vi "think_and_act_2.vi"(8 "error in (no error)":errorcluster, 9 "antState":T1, 10 "pieceOfWorld":T4[][](array[typedef]), 11 "Igor in":refnum<class "Igor.lvclass">) -> (0 "error out":errorcluster, 2 "action":T2, 3 "Igor out":refnum<class "Igor.lvclass">)   [LabVIEW 2015]
doc: "Ant thinks and chooses action\nCreated by Artem Shevelev\nshevelev.pro\nartem@shevelev.pro\nLabVIEW Portal: https://labviewportal.org/memberlist.php?mode=viewprofile&u=2340"
uses:
  ant_base/ant_base.lvclass
  ant_base/actionType_enum.ctl
  ant_base/action_cluster.ctl
  actors/world/typedefs/markValue.ctl
  actors/world/world.lvlib
  actors/world/typedefs/anthillType_enum.ctl
  Igor.lvclass
  az_to_rad/az_to_rad_back.vi
  az_to_rad/az_to_rad_straight.vi
  actors/world/typedefs/markVolume.ctl
  actors/world/typedefs/markValue_cluster.ctl
  actors/world/typedefs/worldCell_cluster.ctl
  ant_base/antState_cluster.ctl
  actors/world/typedefs/amountOfFood.ctl
panel:
  out "Array":i32[][](array[numeric])
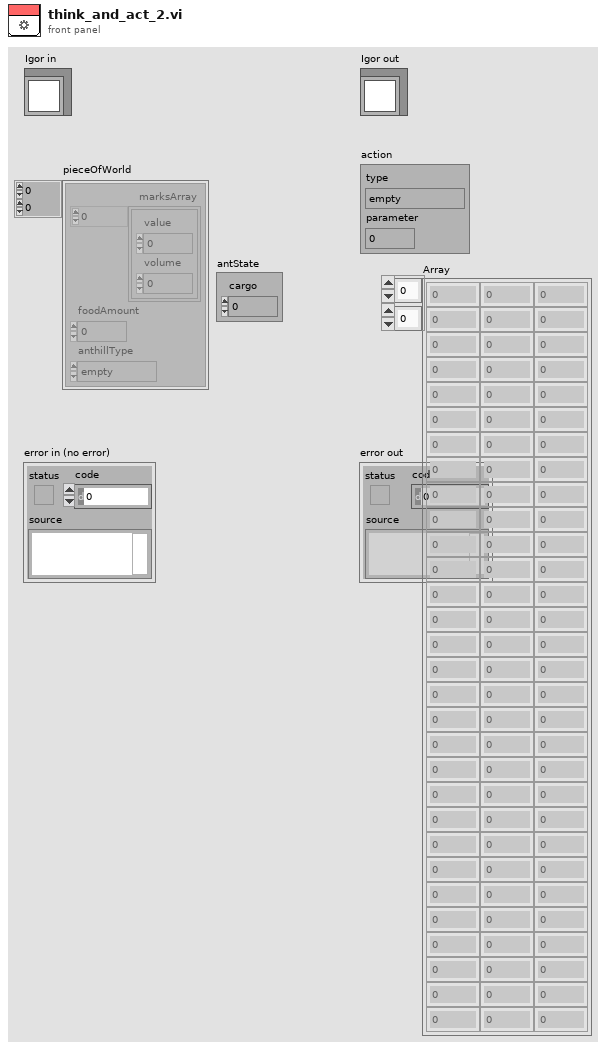
[diagram p1: front panel]
types:
  T1 = typedef "ant_base.lvclass/antState_cluster.ctl" = cluster{"cargo":u8}
  T2 = typedef "ant_base.lvclass/action_cluster.ctl" = cluster{"type":T3, "parameter":dbl}
  T3 = typedef "ant_base.lvclass/actionType_enum.ctl" = enum8{"empty", "move", "take", "put", "mark"}
  T4 = typedef "world.lvlib/worldCell_cluster.ctl" = cluster{"marksArray":T5[], "foodAmount":T8, "anthillType":T9}
  T5 = typedef "world.lvlib/markValue_cluster.ctl" = cluster{"value":T6, "volume":T7}
  T6 = typedef "world.lvlib/markValue.ctl" = u8
  T7 = typedef "world.lvlib/markVolume.ctl" = u16
  T8 = typedef "world.lvlib/amountOfFood.ctl" = i32
  T9 = typedef "world.lvlib/anthillType_enum.ctl" = enum16{"empty", "own", "rival"}
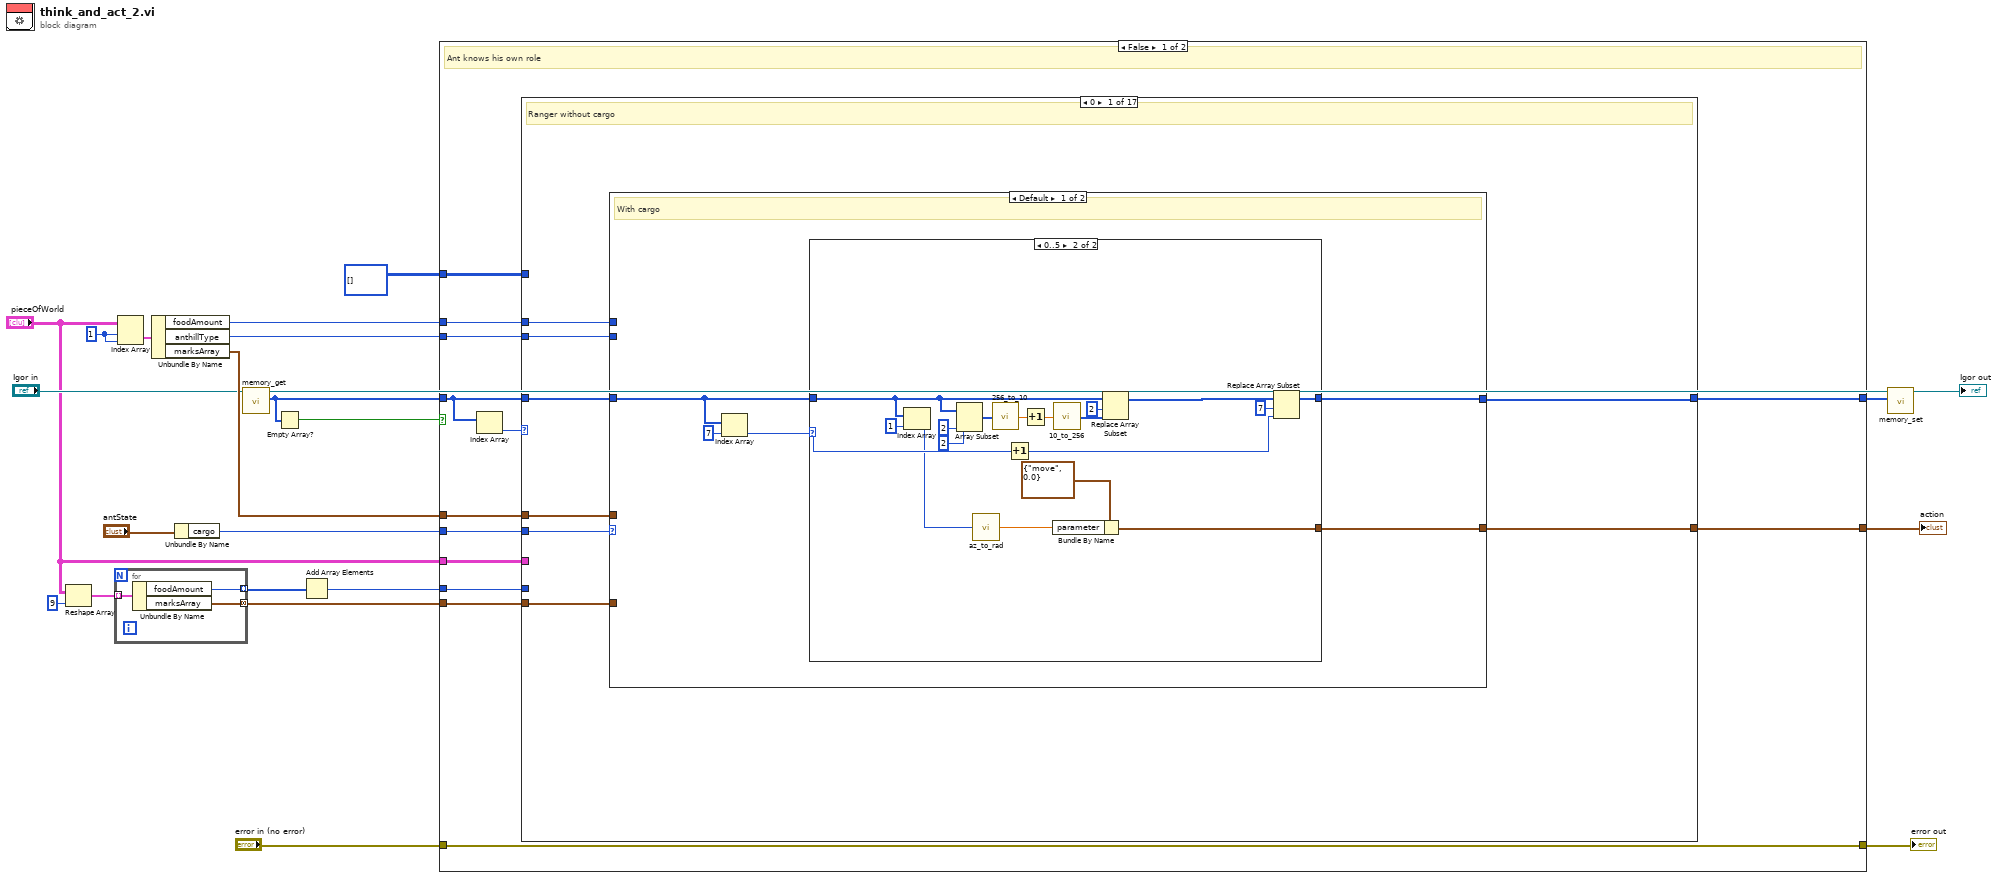
[diagram p0: block diagram]
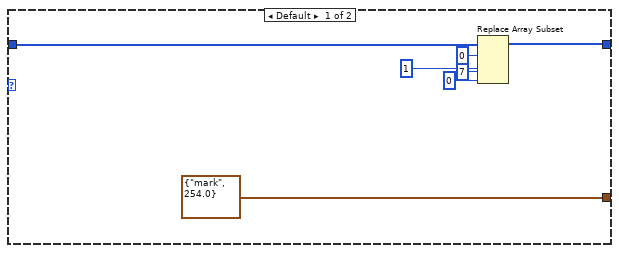
[diagram p2: hidden frame]
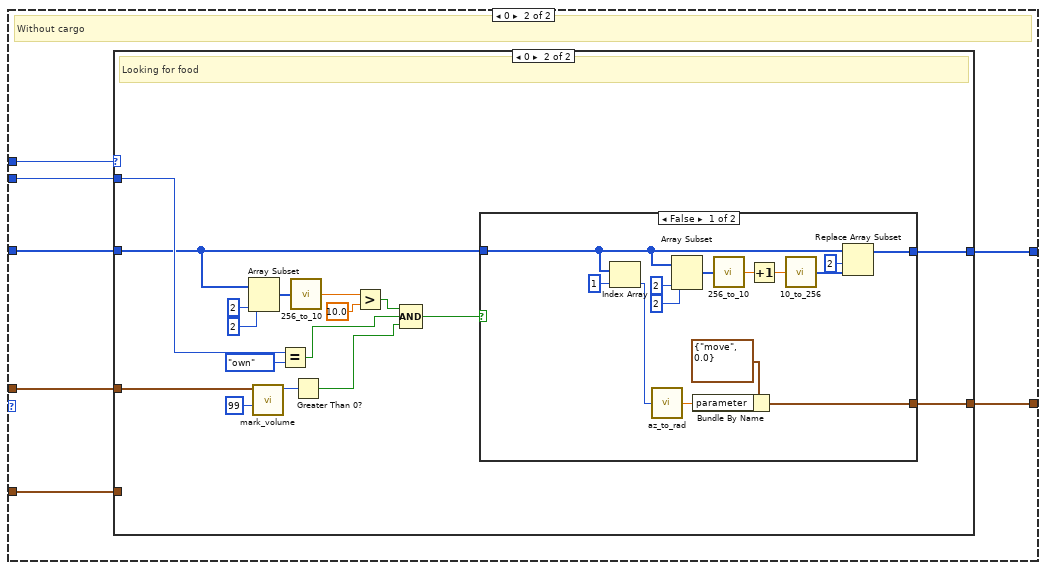
[diagram p3: hidden frame]
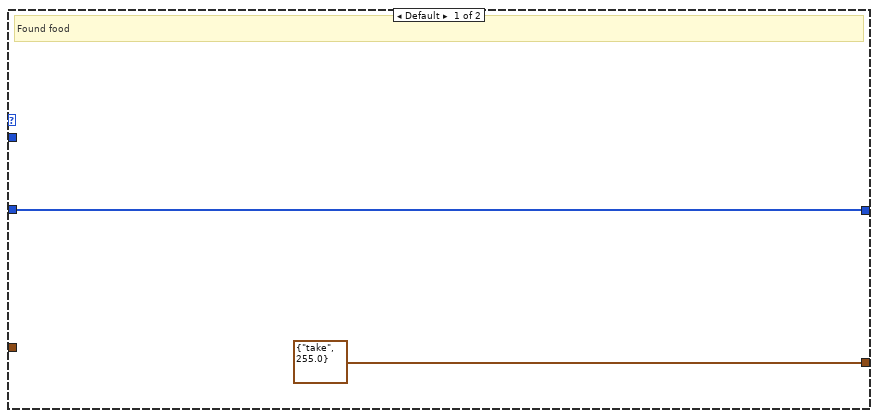
[diagram p4: hidden frame]
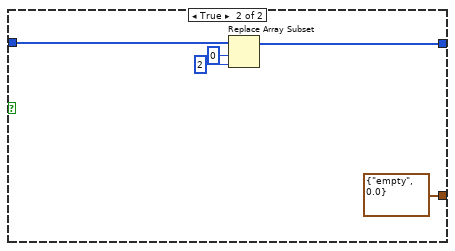
[diagram p5: hidden frame]
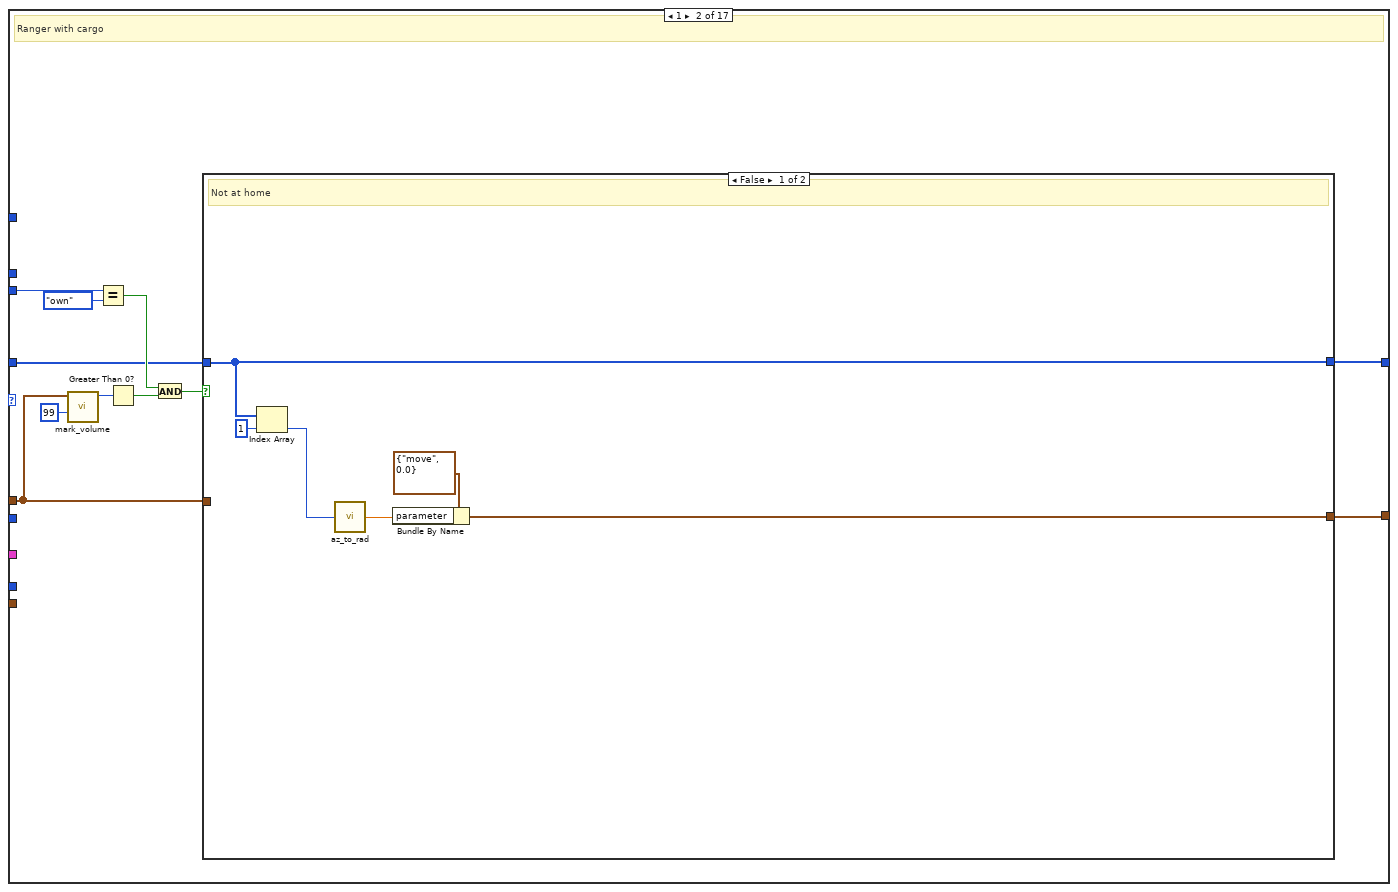
[diagram p6: hidden frame]
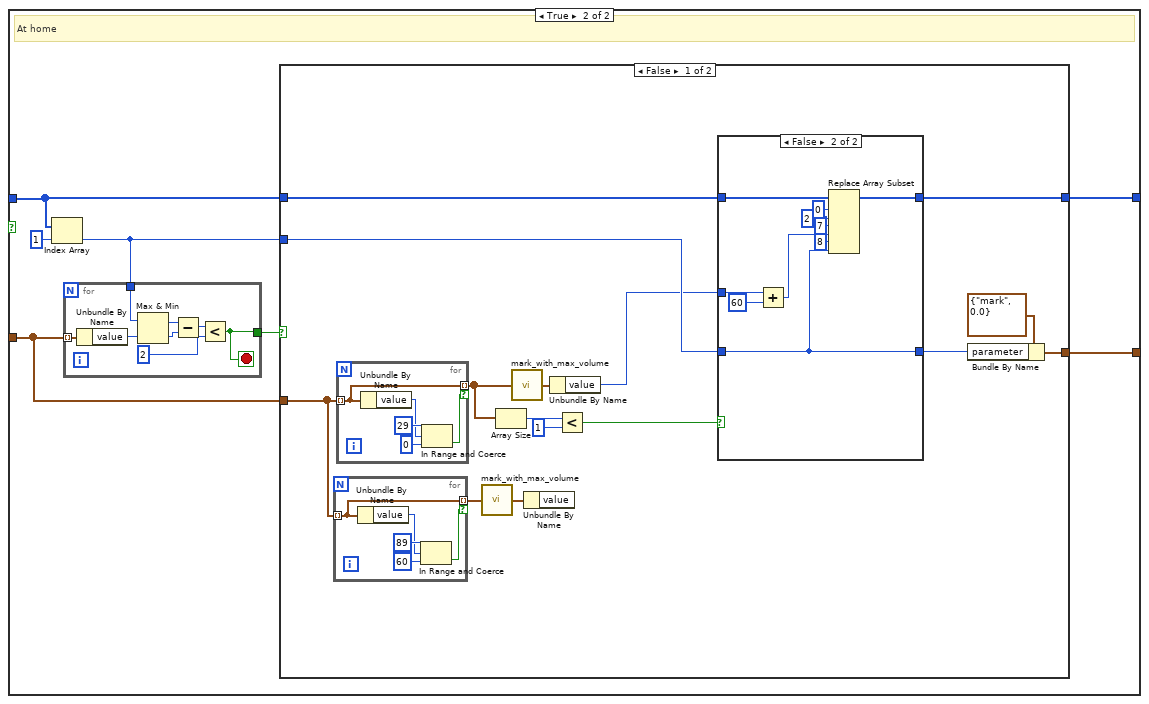
[diagram p7: hidden frame]
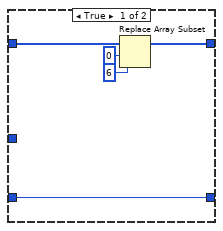
[diagram p8: hidden frame]
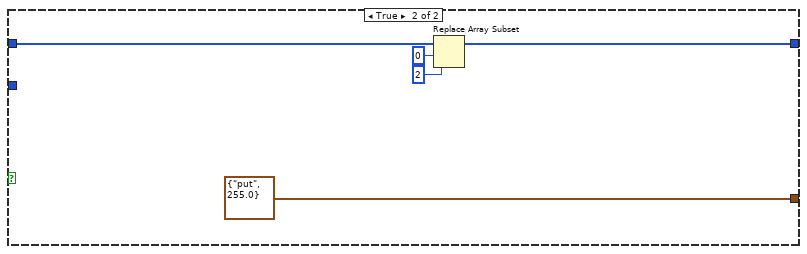
[diagram p9: hidden frame]
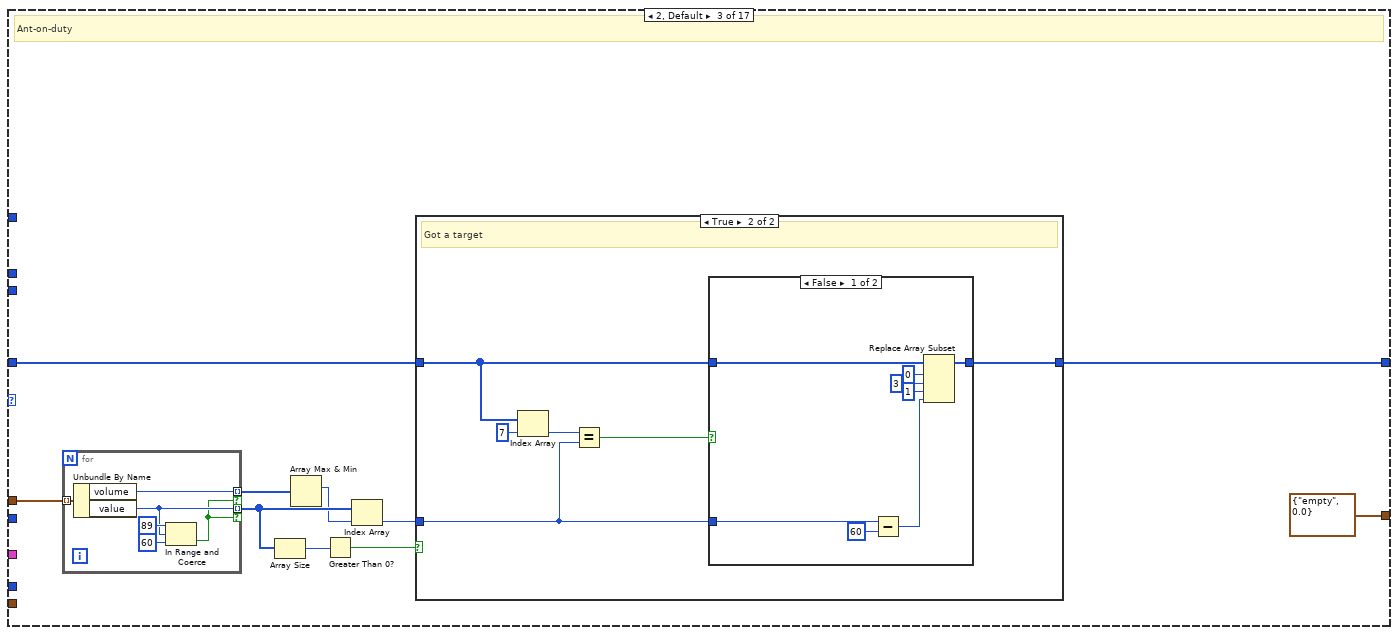
[diagram p10: hidden frame]
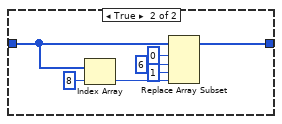
[diagram p12: hidden frame]
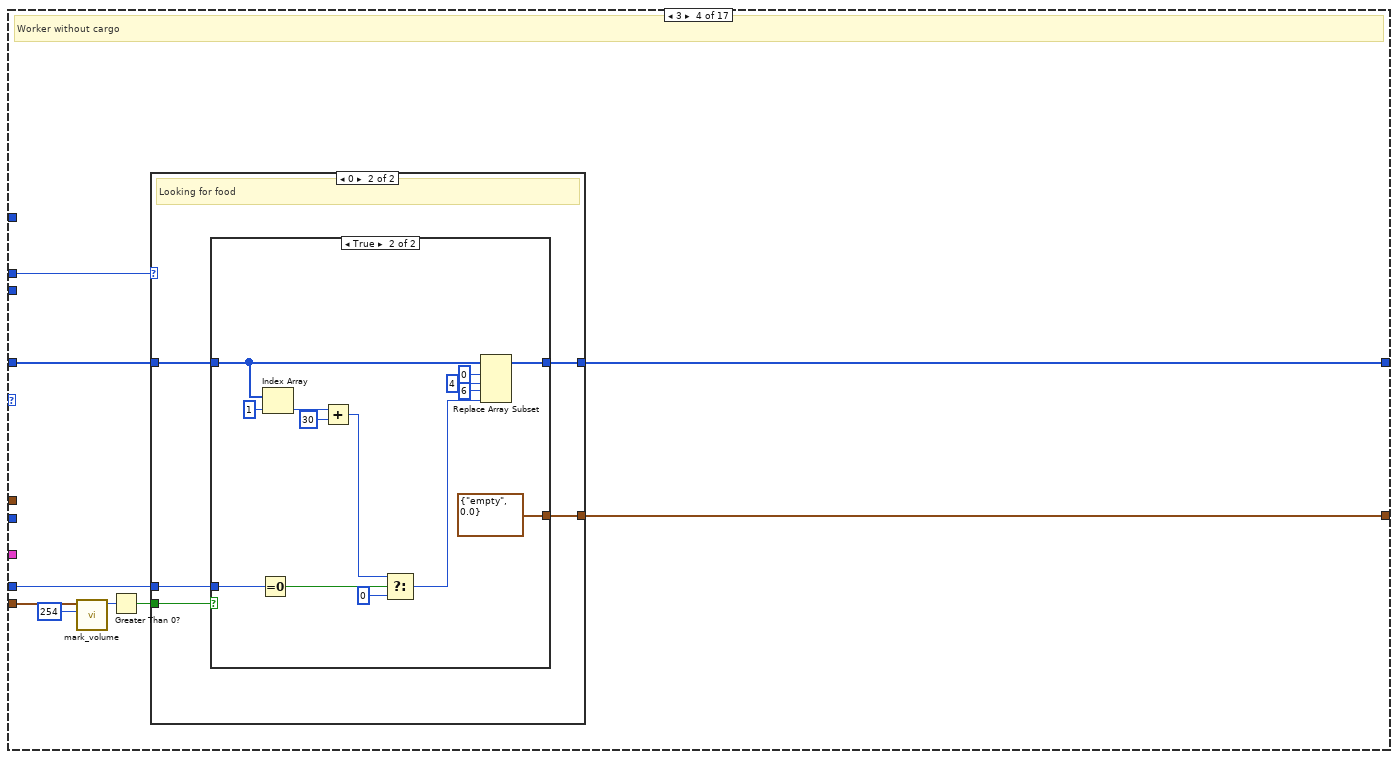
[diagram p13: hidden frame]
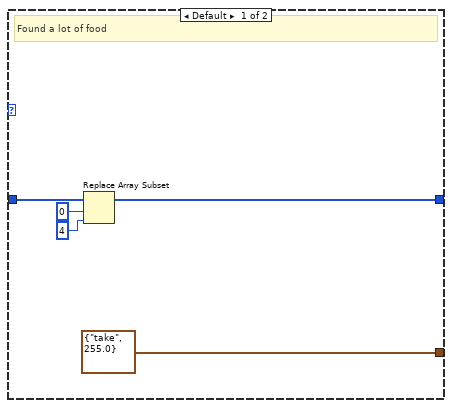
[diagram p14: hidden frame]
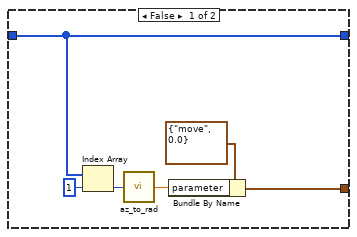
[diagram p15: hidden frame]
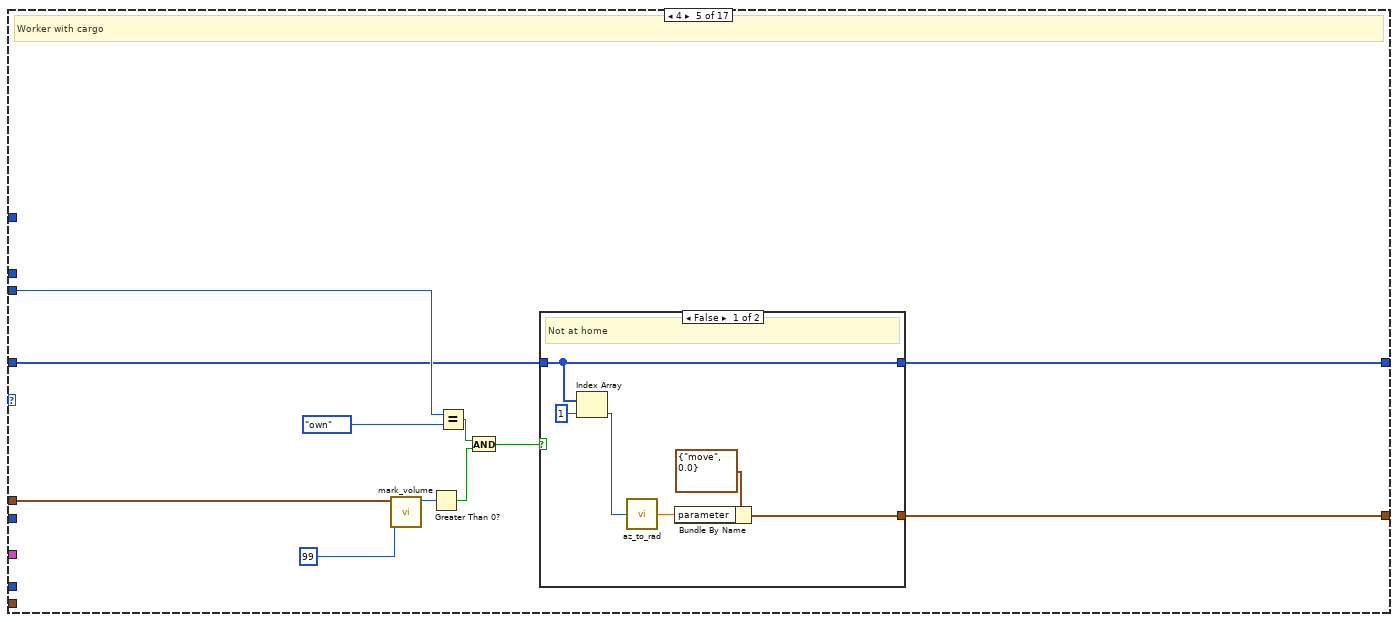
[diagram p16: hidden frame]
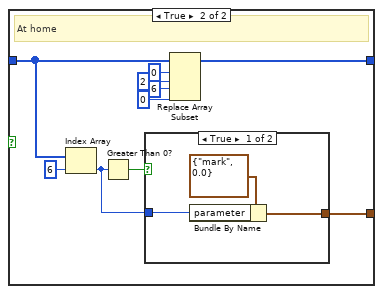
[diagram p17: hidden frame]
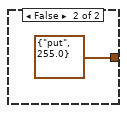
[diagram p18: hidden frame]
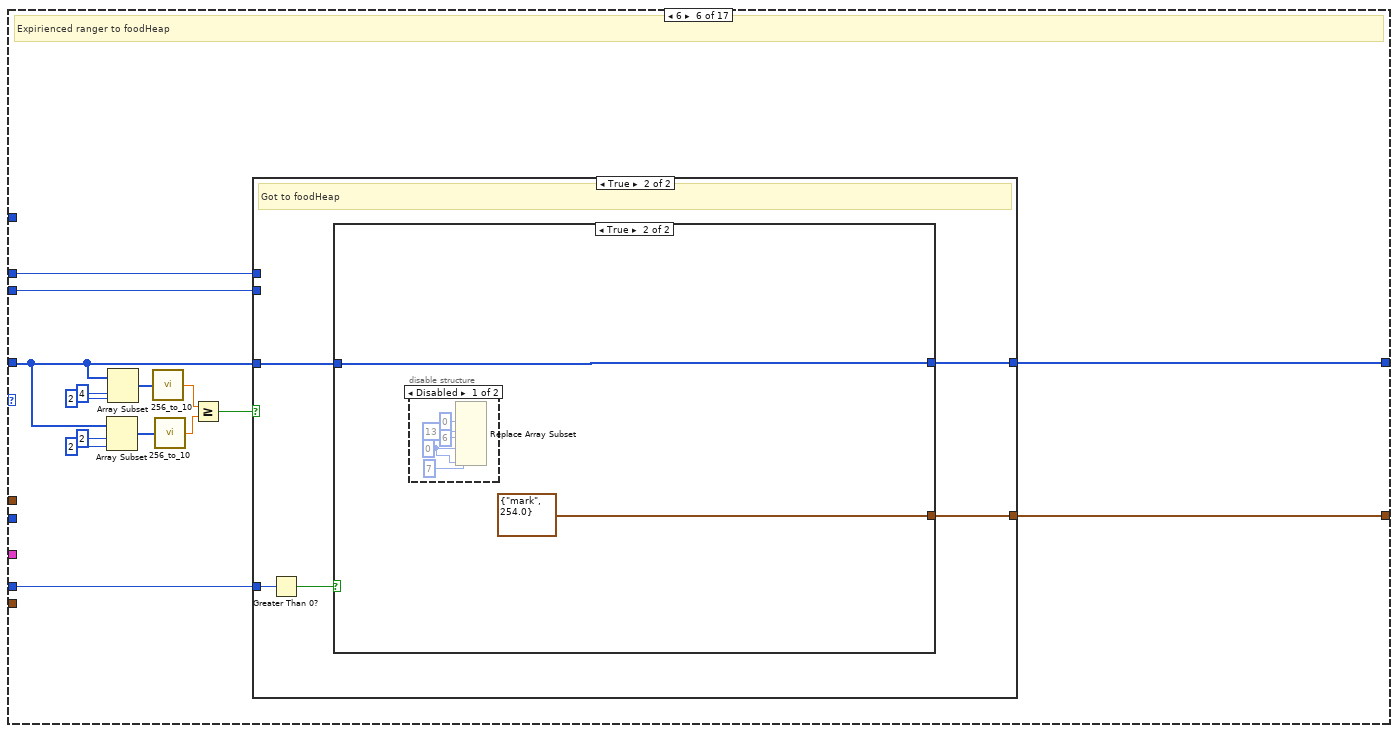
[diagram p19: hidden frame]
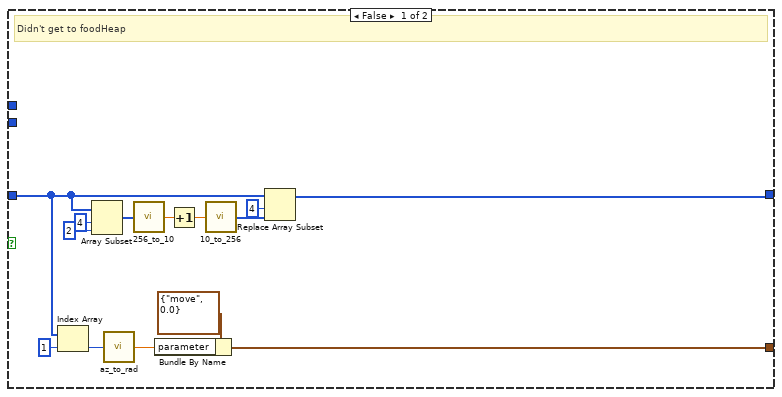
[diagram p20: hidden frame]
diagram:
  w23 = 1 ("index (row)")
  n1 = Reshape Array("pieceOfWorld", 9 ("dimension size")) -> (w10:T4[])
  n2 = for {
    tunnel: w10 -> [w26] mode=indexing
    tunnel: [w25] -> w9 mode=concatenating
    tunnel: [w24] -> w8 mode=indexing
    n3 = Unbundle By Name(w26) -> ("foodAmount"=w24:T8, "marksArray"=w25:T5[])
  }
  n4 = Index Array(array="pieceOfWorld", index (row)=w23, index (col)=w23) -> (element=w22:T4)
  n5 = Unbundle By Name(w22) -> ("foodAmount"=w14:T8, "anthillType"=w13:T9, "marksArray"=w18:T5[])
  n6 = Unbundle By Name("antState") -> ("cargo"=w2:u8)
  n7 = call "memory_get.vi"("ant_base in"="Igor in") -> ("memory"=w15:u8[], "ant_base out"=w5:refnum<class "Igor.lvclass">)  [unwired: 8 in, 1 out]
  n8 = Empty Array?(array=w15) -> (empty?=w16:bool)
  n9 = Add Array Elements(numeric array=w8) -> (sum=w7:T8)
  n10 = case shown="False" w16 {
    tunnel: [w39 w791] -> w21
    tunnel: [w37 w790] -> w20
    tunnel: "error in (no error)" -> [w39 w791]
    tunnel: w18 -> [w34 w786]
    tunnel: w15 -> [w33 w787]
    tunnel: w14 -> [w36 _]
    tunnel: w13 -> [w35 _]
    tunnel: "pieceOfWorld" -> [w32 _]
    tunnel: w9 -> [w31 _]
    tunnel: w7 -> [w30 _]
    tunnel: [w29 w788] -> w4
    tunnel: w2 -> [w28 _]
    tunnel: i32[][] [] -> [w27 _]
    frame False {
      # "Ant knows his own role"
      n11 = Index Array(array=w33) -> (element=w38:u8)  [unwired: 1 in]
      n12 = case shown="0" w38 {
        tunnel: [w47 w133 T2 {"type"=enum."empty", "parameter"=0.0} ("action") w245 w286 w313 w365 w409 T2 {"type"=enum."empty", "parameter"=0.0} ("action") w433 T2 {"type"=enum."empty", "parameter"=0.0} ("action") w525 w548 w575 w612 w637 w685] -> w37
        tunnel: w36 -> [w46 _ _ w239 _ w314 _ _ _ w430 _ _ _ _ w613 _ _]
        tunnel: w35 -> [w44 w132 _ _ w287 w311 w367 _ _ w431 _ _ _ w574 w611 w639 _]
        tunnel: w34 -> [w41 w126 w209 _ w279 _ w359 w400 _ _ w473 _ _ w568 w608 w632 w678]
        tunnel: w33 -> [w45 w128 w201 w246 w285 w315 w366 w410 w427 w435 w487 w524 w547 w570 w614 w638 w684]
        tunnel: w32 -> [_ _ _ _ _ _ _ _ _ _ _ _ _ _ _ _ _]
        tunnel: w31 -> [w43 _ _ w240 _ _ _ _ _ _ _ _ _ _ _ _ _]
        tunnel: w30 -> [_ _ _ w238 _ w310 _ _ _ _ _ _ _ _ w610 _ _]
        tunnel: [w42 w123 w200 w241 w277 w309 w360 w401 w425 w434 w486 w523 w546 w565 w609 w631 w683] -> w29
        tunnel: w28 -> [w40 _ _ _ _ _ _ _ _ w432 _ _ _ _ _ _ _]
        tunnel: w27 -> [_ _ _ _ _ _ _ _ _ _ _ _ _ _ _ _ w679]
        frame 0 {
          # "Ranger without cargo"
          n13 = case shown="Default" w40 {
            tunnel: [w51 w84] -> w47
            tunnel: w46 -> [_ w83]
            tunnel: w45 -> [w50 w82]
            tunnel: w44 -> [_ w81]
            tunnel: w43 -> [_ w80]
            tunnel: [w52 w79] -> w42
            tunnel: w41 -> [_ w78]
            frame Default {
              # "With cargo"
              n14 = Index Array(array=w50, index=7) -> (element=w48:u8)
              n15 = case shown="0..5" w48 {
                selector: w48 -> [_ w72]
                tunnel: [w56 w77] -> w52
                tunnel: w50 -> [w57 w62]
                tunnel: [T2 {"type"=enum."mark", "parameter"=254.0} ("action") w73] -> w51
                frame Default {
                  n16 = Replace Array Subset(array=w57, new element #1=u8 1 ("new element/subarray"), index #1=0 ("index"), new element #2=u8 0 ("new element/subarray"), index #2=7 ("index")) -> (w56:u8[])
                }
                frame 0..5 {
                  n17 = Index Array(array=w62, index=1) -> (element=w61:u8)
                  n18 = Array Subset(array=w62, index=2, length=2) -> (w67:u8[])
                  n19 = call-poly "az_to_rad.vi"("az"=w61) -> ("rad"=w75:dbl)
                  n20 = call "256_to_10.vi"("Array"=w67) -> ("Numeric"=w66:dbl)
                  n21 = Increment(x=w72) -> (x+1=w71:u8)
                  n22 = Increment(x=w66) -> (x+1=w65:dbl)
                  n23 = Bundle By Name(cluster=T2 {"type"=enum."move", "parameter"=0.0} ("action"), "parameter"=w75) -> (w73:T2)
                  n24 = call "10_to_256.vi"("Decimal"=w65) -> ("256"=w64:u8[])
                  n25 = Replace Array Subset(array=w62, new element=w64, index=2) -> (w60:u8[])
                  n26 = Replace Array Subset(array=w60, new element=w71, index=7) -> (w77:u8[])
                }
              }
            }
            frame 0 {
              # "Without cargo"
              n27 = case shown="0" w83 {
                tunnel: [T2 {"type"=enum."take", "parameter"=255.0} ("action") w103] -> w84
                tunnel: w82 -> [w85 w93]
                tunnel: w81 -> [_ w97]
                tunnel: w80 -> [_ _]
                tunnel: [w85 w102] -> w79
                tunnel: w78 -> [_ w98]
                frame Default {
                  # "Found food"
                }
                frame 0 {
                  # "Looking for food"
                  n28 = Array Subset(array=w93, index=2, length=2) -> (w94:u8[])
                  n29 = call "mark_volume.vi"("element"=T6 99, "marksArray"=w98) -> ("volume"=w99:T7)  [unwired: 9 in]
                  n30 = Equal?(x=w97, y=anthillType_enum."own") -> (x = y?=w89:bool)
                  n31 = call "256_to_10.vi"("Array"=w94) -> ("Numeric"=w92:dbl)
                  n32 = Greater Than 0?(x=w99) -> (x > 0?=w88:bool)
                  n33 = Greater?(x=w92, y=10.0) -> (0:w90:bool)
                  n34 = Compound Arithmetic op=AND(w90, w89, w88) -> (w87:bool)
                  n35 = case shown="False" w87 {
                    tunnel: [w117 T2 {"type"=enum."empty", "parameter"=0.0} ("action")] -> w103
                    tunnel: [w105 w121] -> w102
                    tunnel: w93 -> [w104 w122]
                    frame False {
                      n36 = Index Array(array=w104, index=1) -> (element=w107:u8)
                      n37 = call-poly "az_to_rad.vi"("az"=w107) -> ("rad"=w108:dbl)
                      n38 = Array Subset(array=w104, index=2, length=2) -> (w112:u8[])
                      n39 = Bundle By Name(cluster=T2 {"type"=enum."move", "parameter"=0.0} ("action"), "parameter"=w108) -> (w117:T2)
                      n40 = call "256_to_10.vi"("Array"=w112) -> ("Numeric"=w111:dbl)
                      n41 = Increment(x=w111) -> (x+1=w110:dbl)
                      n42 = call "10_to_256.vi"("Decimal"=w110) -> ("256"=w109:u8[])
                      n43 = Replace Array Subset(array=w104, new element=w109, index=2) -> (w105:u8[])
                    }
                    frame True {
                      n44 = Replace Array Subset(array=w122, new element=u8 2 ("new element/subarray"), index=0) -> (w121:u8[])
                    }
                  }
                }
              }
            }
          }
        }
        frame 1 {
          # "Ranger with cargo"
          n45 = call "mark_volume.vi"("element"=T6 99, "marksArray"=w126) -> ("volume"=w125:T7)  [unwired: 9 in]
          n46 = Equal?(x=w132, y=anthillType_enum."own") -> (x = y?=w130:bool)
          n47 = Greater Than 0?(x=w125) -> (x > 0?=w124:bool)
          n48 = And(x=w130, y=w124) -> (x .and. y?=w129:bool)
          n49 = case shown="False" w129 {
            tunnel: [w138 w145] -> w133
            tunnel: w126 -> [_ w140]
            tunnel: w128 -> [w134 w143]
            tunnel: [w134 w141] -> w123
            frame False {
              # "Not at home"
              n50 = Index Array(array=w134, index=1) -> (element=w135:u8)
              n51 = call-poly "az_to_rad.vi"("az"=w135) -> ("rad"=w137:dbl)
              n52 = Bundle By Name(cluster=T2 {"type"=enum."move", "parameter"=0.0} ("action"), "parameter"=w137) -> (w138:T2)
            }
            frame True {
              # "At home"
              n53 = Index Array(array=w143, index=1) -> (element=w142:u8)
              n54 = for {
                tunnel: w140 -> [w199] mode=indexing
                tunnel: w142 -> [w193]
                tunnel: [w192] -> w146
                stop <- w192 stop-if-true
                n55 = Unbundle By Name(w199) -> ("value"=w194:T6)
                n56 = Max & Min(x=w193, y=w194) -> (max(x,y)=w198:T6, min(x,y)=w197:u8)
                n57 = Subtract(x=w198, y=w197) -> (x-y=w196:T6)
                n58 = Less?(x=w196, y=T6 2) -> (x < y?=w192:bool)
              }
              n59 = case shown="False" w146 {
                tunnel: [w161 T2 {"type"=enum."put", "parameter"=255.0} ("action")] -> w145
                tunnel: w142 -> [w153 _]
                tunnel: w143 -> [w159 w190]
                tunnel: [w158 w189] -> w141
                tunnel: w140 -> [w156 _]
                frame False {
                  n60 = for {
                    tunnel: w156 -> [w177] mode=indexing
                    tunnel: [w177] -> w157 mode=indexing if=w178
                    n61 = Unbundle By Name(w177) -> ("value"=w179:T6)
                    n62 = In Range and Coerce(upper limit=T6 89, x=w179, lower limit=T6 60) -> (In Range?=w178:bool)  [unwired: 1 out]
                  }
                  n63 = for {
                    tunnel: w156 -> [w182] mode=indexing
                    tunnel: [w182] -> w151 mode=indexing if=w183
                    n64 = Unbundle By Name(w182) -> ("value"=w184:T6)
                    n65 = In Range and Coerce(upper limit=T6 29, x=w184, lower limit=T6 0) -> (In Range?=w183:bool)  [unwired: 1 out]
                  }
                  n66 = call "mark_with_max_volume.vi"("marksArray"=w157) -> ("markValue"=w155:T5)
                  n67 = Array Size(array=w151) -> (size(s)=w150:i32)
                  n68 = call "mark_with_max_volume.vi"("marksArray"=w151) -> ("markValue"=w154:T5)
                  n69 = Unbundle By Name(w155) -> ()  [unwired: 1 out]
                  n70 = Unbundle By Name(w154) -> ("value"=w152:T6)
                  n71 = Less?(x=w150, y=1) -> (x < y?=w148:bool)
                  n72 = case shown="False" w148 {
                    tunnel: w159 -> [w166 w176]
                    tunnel: [w164 w174] -> w158
                    tunnel: w153 -> [w162 w167]
                    tunnel: w152 -> [_ w170]
                    tunnel: [w162 w167] -> w147
                    frame True {
                      n73 = Replace Array Subset(array=w166, new element=u8 6 ("new element/subarray"), index=0) -> (w164:u8[])
                    }
                    frame False {
                      n74 = Add(x=w170, y=T6 60) -> (x+y=w168:T6)
                      n75 = Replace Array Subset(array=w176, new element #1=u8 2 ("new element/subarray"), index #1=0 ("index"), new element #2=w168, index #2=7 ("index"), new element #3=w167, index #3=8 ("index")) -> (w174:u8[])
                    }
                  }
                  n76 = Bundle By Name(cluster=T2 {"type"=enum."mark", "parameter"=0.0} ("action"), "parameter"=w147) -> (w161:T2)
                }
                frame True {
                  n77 = Replace Array Subset(array=w190, new element=u8 2 ("new element/subarray"), index=0) -> (w189:u8[])
                }
              }
            }
          }
        }
        frame 2, Default {
          # "Ant-on-duty"
          n78 = for {
            tunnel: w209 -> [w213] mode=indexing
            tunnel: [w211] -> w205 mode=indexing if=w210
            tunnel: [w212] -> w207 mode=indexing if=w210
            n79 = Unbundle By Name(w213) -> ("volume"=w212:T7, "value"=w211:T6)
            n80 = In Range and Coerce(upper limit=T6 89, x=w211, lower limit=T6 60) -> (In Range?=w210:bool)  [unwired: 1 out]
          }
          n81 = Array Size(array=w205) -> (size(s)=w204:i32)
          n82 = Array Max & Min(array=w207) -> (max index (indices)=w202:i32)  [unwired: 3 out]
          n83 = Greater Than 0?(x=w204) -> (x > 0?=w203:bool)
          n84 = Index Array(array=w205, index=w202) -> (element=w206:T6)
          n85 = case shown="True" w203 {
            tunnel: w206 -> [_ w218]
            tunnel: w201 -> [w216 w221]
            tunnel: [w216 w222] -> w200
            frame False {
              # "Expecting a target"
            }
            frame True {
              # "Got a target"
              n86 = Index Array(array=w221, index=7) -> (element=w219:u8)
              n87 = Equal?(x=w219, y=w218) -> (x = y?=w217:bool)
              n88 = case shown="False" w217 {
                tunnel: w218 -> [w230 _]
                tunnel: w221 -> [w228 w232]
                tunnel: [w223 w234] -> w222
                frame False {
                  n89 = Subtract(x=w230, y=T6 60) -> (x-y=w224:T6)
                  n90 = Replace Array Subset(array=w228, new element #1=u8 3 ("new element/subarray"), index #1=0 ("index"), new element #2=w224, index #2=1 ("index")) -> (w223:u8[])
                }
                frame True {
                  n91 = Index Array(array=w232, index=8) -> (element=w231:u8)
                  n92 = Replace Array Subset(array=w232, new element #1=u8 6 ("new element/subarray"), index #1=0 ("index"), new element #2=w231, index #2=1 ("index")) -> (w234:u8[])
                }
              }
            }
          }
        }
        frame 3 {
          # "Worker without cargo"
          n93 = call "mark_volume.vi"("element"=T6 254, "marksArray"=w240) -> ("volume"=w243:T7)  [unwired: 9 in]
          n94 = Greater Than 0?(x=w243) -> (x > 0?=w242:bool)
          n95 = case shown="0" w239 {
            tunnel: [T2 {"type"=enum."take", "parameter"=255.0} ("action") w256] -> w245
            tunnel: w246 -> [w250 w254]
            tunnel: w242 -> [_ w255]
            tunnel: [w247 w253] -> w241
            tunnel: w238 -> [_ w252]
            frame Default {
              # "Found a lot of food"
              n96 = Replace Array Subset(array=w250, new element=4 ("index"), index=0) -> (w247:u8[])
            }
            frame 0 {
              # "Looking for food"
              n97 = case shown="True" w255 {
                tunnel: [w261 T2 {"type"=enum."empty", "parameter"=0.0} ("action")] -> w256
                tunnel: w254 -> [w257 w269]
                tunnel: [w257 w268] -> w253
                tunnel: w252 -> [_ w267]
                frame False {
                  n98 = Index Array(array=w257, index=1) -> (element=w258:u8)
                  n99 = call-poly "az_to_rad.vi"("az"=w258) -> ("rad"=w260:dbl)
                  n100 = Bundle By Name(cluster=T2 {"type"=enum."move", "parameter"=0.0} ("action"), "parameter"=w260) -> (w261:T2)
                }
                frame True {
                  n101 = Equal To 0?(x=w267) -> (x = 0?=w266:bool)
                  n102 = Index Array(array=w269, index=1) -> (element=w271:u8)
                  n103 = Add(x=w271, y=u8 30) -> (x+y=w265:u8)
                  n104 = Select(t=w265, s=w266, f=u8 0) -> (s? t:f=w263:u8)
                  n105 = Replace Array Subset(array=w269, new element #1=u8 4 ("new element/subarray"), index #1=0 ("index"), new element #2=w263, index #2=6 ("index")) -> (w268:u8[])
                }
              }
            }
          }
        }
        frame 4 {
          # "Worker with cargo"
          n106 = call "mark_volume.vi"("element"=T6 99, "marksArray"=w279) -> ("volume"=w280:T7)  [unwired: 9 in]
          n107 = Greater Than 0?(x=w280) -> (x > 0?=w278:bool)
          n108 = Equal?(x=w287, y=anthillType_enum."own") -> (x = y?=w283:bool)
          n109 = And(x=w283, y=w278) -> (x .and. y?=w282:bool)
          n110 = case shown="False" w282 {
            tunnel: [w292 w300] -> w286
            tunnel: w285 -> [w288 w299]
            tunnel: [w288 w294] -> w277
            frame False {
              # "Not at home"
              n111 = Index Array(array=w288, index=1) -> (element=w289:u8)
              n112 = call-poly "az_to_rad.vi"("az"=w289) -> ("rad"=w291:dbl)
              n113 = Bundle By Name(cluster=T2 {"type"=enum."move", "parameter"=0.0} ("action"), "parameter"=w291) -> (w292:T2)
            }
            frame True {
              # "At home"
              n114 = Index Array(array=w299, index=6) -> (element=w301:u8)
              n115 = Greater Than 0?(x=w301) -> (x > 0?=w302:bool)
              n116 = case shown="True" w302 {
                tunnel: w301 -> [w305 _]
                tunnel: [w304 T2 {"type"=enum."put", "parameter"=255.0} ("action")] -> w300
                frame True {
                  n117 = Bundle By Name(cluster=T2 {"type"=enum."mark", "parameter"=0.0} ("action"), "parameter"=w305) -> (w304:T2)
                }
                frame False {
                }
              }
              n118 = Replace Array Subset(array=w299, new element #1=u8 2 ("y"), index #1=0 ("index"), new element #2=u8 0 ("new element/subarray"), index #2=6 ("index")) -> (w294:u8[])
            }
          }
        }
        frame 6 {
          # "Expirienced ranger to foodHeap"
          n119 = Array Subset(array=w315, index=2, length=2 ("index")) -> (w318:u8[])
          n120 = Array Subset(array=w315, index=4, length=2) -> (w320:u8[])
          n121 = call "256_to_10.vi"("Array"=w320) -> ("Numeric"=w317:dbl)
          n122 = call "256_to_10.vi"("Array"=w318) -> ("Numeric"=w308:dbl)
          n123 = Greater Or Equal?(x=w317, y=w308) -> (x >= y?=w316:bool)
          n124 = case shown="True" w316 {
            tunnel: [w323 w339] -> w309
            tunnel: w315 -> [w325 w340]
            tunnel: w314 -> [_ _]
            tunnel: [w335 w341] -> w313
            tunnel: w311 -> [_ _]
            tunnel: w310 -> [_ w338]
            frame False {
              # "Didn't get to foodHeap"
              n125 = Index Array(array=w325, index=1) -> (element=w324:u8)
              n126 = Array Subset(array=w325, index=4, length=2) -> (w331:u8[])
              n127 = call-poly "az_to_rad.vi"("az"=w324) -> ("rad"=w327:dbl)
              n128 = call "256_to_10.vi"("Array"=w331) -> ("Numeric"=w330:dbl)
              n129 = Bundle By Name(cluster=T2 {"type"=enum."move", "parameter"=0.0} ("action"), "parameter"=w327) -> (w335:T2)
              n130 = Increment(x=w330) -> (x+1=w329:dbl)
              n131 = call "10_to_256.vi"("Decimal"=w329) -> ("256"=w328:u8[])
              n132 = Replace Array Subset(array=w325, new element=w328, index=4) -> (w323:u8[])
            }
            frame True {
              # "Got to foodHeap"
              n133 = Greater Than 0?(x=w338) -> (x > 0?=w337:bool)
              n134 = case shown="True" w337 {
                tunnel: [T2 {"type"=enum."mark", "parameter"=254.0} ("action") T2 {"type"=enum."mark", "parameter"=254.0} ("action")] -> w341
                tunnel: w340 -> [w344 w352]
                tunnel: [w343 w352] -> w339
                frame False {
                  n135 = Index Array(array=w344, index=1) -> (element=w345:u8)
                  n136 = Add(x=w345, y=u8 30) -> (x+y=w342:u8)
                  n137 = Replace Array Subset(array=w344, new element #1=u8 7 ("new element/subarray"), index #1=0 ("index"), new element #2=w342, index #2=6 ("index")) -> (w343:u8[])
                }
                frame True {
                  n138 = disable-structure shown="Disabled" {
                    frame Disabled {
                      w354 = 0 ("index")
                      n139 = Replace Array Subset(new element #1=u8 13 ("new element/subarray"), index #1=0 ("index"), new element #2=w354, index #2=6 ("index"), new element #3=w354, index #3=7 ("index")) -> ()  [unwired: 1 in, 1 out]
                    }
                    frame Enabled {
                    }
                  }
                }
              }
            }
          }
        }
        frame 7 {
          # "Expirienced ranger from foodHeap"
          n140 = call "mark_volume.vi"("element"=T6 99, "marksArray"=w359) -> ("volume"=w362:T7)  [unwired: 9 in]
          n141 = Equal?(x=w367, y=anthillType_enum."own") -> (x = y?=w368:bool)
          n142 = Greater Than 0?(x=w362) -> (x > 0?=w361:bool)
          n143 = And(x=w368, y=w361) -> (x .and. y?=w364:bool)
          n144 = case shown="True" w364 {
            tunnel: [w374 w384] -> w365
            tunnel: w366 -> [w370 w381]
            tunnel: [w370 w383] -> w360
            tunnel: w359 -> [_ w382]
            frame False {
              # "Not at home"
              n145 = Index Array(array=w370, index=1) -> (element=w371:u8)
              n146 = call-poly "az_to_rad.vi"("az"=w371) -> ("rad"=w373:dbl)
              n147 = Bundle By Name(cluster=T2 {"type"=enum."move", "parameter"=0.0} ("action"), "parameter"=w373) -> (w374:T2)
            }
            frame True {
              # "At home"
              n148 = Index Array(array=w381, index=1) -> (element=w379:u8)
              n149 = Add(x=w379, y=u8 30) -> (x+y=w377:u8)
              n150 = call "mark_volume.vi"("element"=w377, "marksArray"=w382) -> ("volume"=w376:T7)  [unwired: 9 in]
              n151 = case shown="0" w376 {
                selector: w376 -> [w386 _]
                tunnel: [w390 T2 {"type"=enum."put", "parameter"=255.0} ("action")] -> w384
                tunnel: w381 -> [w387 w397]
                tunnel: [w385 w395] -> w383
                frame Default {
                  n152 = Bundle By Name(cluster=T2 {"type"=enum."empty", "parameter"=0.0} ("action"), "parameter"=w386) -> (w390:T2)
                  n153 = Replace Array Subset(array=w387, new element=u8 2 ("new element/subarray"), index=0) -> (w385:u8[])
                }
                frame 0 {
                  w392 = u8 0 ("new element/subarray")
                  n154 = Replace Array Subset(array=w397, new element #1=u8 6 ("new element/subarray"), index #1=0 ("index"), new element #2=w392, index #2=4 ("index"), new element #3=w392, index #3=5 ("index")) -> (w395:u8[])
                }
              }
            }
          }
        }
        frame 8 {
          n155 = Index Array(array=w410, index=1) -> (element=w406:u8)
          n156 = Add(x=w406, y=u8 60) -> (x+y=w412:u8)
          n157 = Add(x=w406, y=u8 30) -> (x+y=w407:u8)
          n158 = call "mark_volume.vi"("element"=w412, "marksArray"=w400) -> ("volume"=w414:T7)  [unwired: 9 in]
          n159 = call "mark_volume.vi"("element"=w407, "marksArray"=w400) -> ("volume"=w405:T7)  [unwired: 9 in]
          n160 = Greater Than 0?(x=w414) -> (x > 0?=w403:bool)
          n161 = Equal To 0?(x=w405) -> (x = 0?=w404:bool)
          n162 = And(x=w403, y=w404) -> (x .and. y?=w402:bool)
          n163 = case shown="False" w402 {
            tunnel: w410 -> [w416 w420]
            tunnel: [T2 {"type"=enum."empty", "parameter"=0.0} ("action") w421] -> w409
            tunnel: w406 -> [_ w419]
            tunnel: [w416 w417] -> w401
            frame False {
            }
            frame True {
              n164 = call-poly "az_to_rad.vi"("az"=w419) -> ("rad"=w418:dbl)
              n165 = Replace Array Subset(array=w420, new element=6 ("index"), index=0) -> (w417:u8[])
              n166 = Bundle By Name(cluster=T2 {"type"=enum."empty", "parameter"=0.0} ("action"), "parameter"=w418) -> (w421:T2)
            }
          }
        }
        frame 9 {
          # "Pause"
          n167 = Replace Array Subset(array=w427, new element=3 ("index"), index=0) -> (w425:u8[])
        }
        frame 10 {
          # "If number of ants less than 32"
          n168 = Array Size(array=w435) -> (size(s)=w436:i32)
          n169 = case shown="2, Default" w436 {
            tunnel: w435 -> [w446 w450]
            tunnel: [w445 w450] -> w434
            tunnel: [w437 w451] -> w433
            tunnel: w432 -> [_ w449]
            tunnel: w431 -> [_ w448]
            tunnel: w430 -> [_ w447]
            frame 1 {
              n170 = Random Number (0-1)() -> (number: 0 to 1=w444:dbl)
              n171 = Multiply(x=w444, y=29.0) -> (x*y=w442:dbl)
              n172 = Round To Nearest(number=w442) -> (nearest integer value=w441:dbl)
              n173 = To Unsigned Byte Integer(number=w441) -> (unsigned 8bit integer=w439:u8)
              n174 = Insert Into Array(array=w446, new element=w439) -> (w445:u8[])  [unwired: 1 in]
              n175 = call-poly "az_to_rad.vi"("az"=w439) -> ("rad"=w440:dbl)
              n176 = Bundle By Name(cluster=T2 {"type"=enum."move", "parameter"=0.0} ("action"), "parameter"=w440) -> (w437:T2)
            }
            frame 2, Default {
              n177 = case shown="Default" w449 {
                tunnel: [w454 w465] -> w451
                tunnel: w450 -> [w452 w464]
                tunnel: w448 -> [w455 _]
                tunnel: w447 -> [w453 w463]
                frame Default {
                  n178 = case shown="\"empty\", Default" w455 {
                    tunnel: [w460 T2 {"type"=enum."put", "parameter"=255.0} ("action")] -> w454
                    tunnel: w453 -> [_ _]
                    tunnel: w452 -> [w461 _]
                    frame "empty", Default {
                      n179 = Index Array(array=w461, index=1) -> (element=w456:u8)
                      n180 = call-poly "az_to_rad.vi"("az"=w456) -> ("rad"=w459:dbl)
                      n181 = Bundle By Name(cluster=T2 {"type"=enum."move", "parameter"=0.0} ("action"), "parameter"=w459) -> (w460:T2)
                    }
                    frame "own" {
                    }
                  }
                }
                frame 0 {
                  n182 = case shown="Default" w463 {
                    tunnel: [T2 {"type"=enum."take", "parameter"=255.0} ("action") w470] -> w465
                    tunnel: w464 -> [_ w469]
                    frame Default {
                    }
                    frame 0 {
                      n183 = Index Array(array=w469, index=1) -> (element=w467:u8)
                      n184 = call-poly "az_to_rad.vi"("az"=w467) -> ("rad"=w472:dbl)
                      n185 = Bundle By Name(cluster=T2 {"type"=enum."move", "parameter"=0.0} ("action"), "parameter"=w472) -> (w470:T2)
                    }
                  }
                }
              }
            }
          }
        }
        frame 11 {
          # "Helper"
          n186 = for {
            tunnel: w473 -> [w494] mode=indexing
            tunnel: [w494] -> w483 mode=indexing if=w495
            n187 = Unbundle By Name(w494) -> ("value"=w496:T6)
            n188 = In Range and Coerce(upper limit=T6 89, x=w496, lower limit=T6 60) -> (In Range?=w495:bool)  [unwired: 1 out]
          }
          n189 = for {
            tunnel: w473 -> [w499] mode=indexing
            tunnel: [w499] -> w484 mode=indexing if=w500
            n190 = Unbundle By Name(w499) -> ("value"=w501:T6)
            n191 = In Range and Coerce(upper limit=T6 29, x=w501, lower limit=T6 0) -> (In Range?=w500:bool)  [unwired: 1 out]
          }
          n192 = call "mark_with_max_volume.vi"("marksArray"=w483) -> ("markValue"=w482:T5)
          n193 = call "mark_with_max_volume.vi"("marksArray"=w484) -> ("markValue"=w481:T5)
          n194 = Unbundle By Name(w481) -> ("value"=w477:T6)
          n195 = Unbundle By Name(w482) -> ("value"=w480:T6)
          n196 = for {
            tunnel: w473 -> [w507] mode=indexing
            tunnel: [w505] -> w491 mode=indexing if=w504
            tunnel: [w506] -> w493 mode=indexing if=w504
            n197 = Unbundle By Name(w507) -> ("volume"=w506:T7, "value"=w505:T6)
            n198 = In Range and Coerce(upper limit=T6 89, x=w505, lower limit=T6 60) -> (In Range?=w504:bool)  [unwired: 1 out]
          }
          n199 = Equal To 0?(x=w477) -> (x = 0?=w476:bool)
          n200 = Equal?(x=w477, y=w480) -> (x = y?=w475:bool)
          n201 = Or(x=w476, y=w475) -> (x .or. y?=w474:bool)
          n202 = Select(t=u8 8 ("new element/subarray"), s=w474, f=u8 11 ("new element/subarray")) -> ()  [unwired: 1 out]
          n203 = Array Size(array=w491) -> (size(s)=w490:i32)
          n204 = Array Max & Min(array=w493) -> (max index (indices)=w488:i32)  [unwired: 3 out]
          n205 = Greater Than 0?(x=w490) -> (x > 0?=w489:bool)
          n206 = Index Array(array=w491, index=w488) -> (element=w492:T6)
          n207 = case shown="True" w489 {
            tunnel: w492 -> [_ w518]
            tunnel: w487 -> [w510 w516]
            tunnel: [w510 w511] -> w486
            frame False {
              # "Expecting a target"
            }
            frame True {
              # "Got a target"
              n208 = Subtract(x=w518, y=T6 60) -> (x-y=w512:T6)
              n209 = Replace Array Subset(array=w516, new element #1=u8 3 ("new element/subarray"), index #1=0 ("index"), new element #2=w512, index #2=1 ("index")) -> (w511:u8[])
            }
          }
        }
        frame 12 {
          # "Ranger without cargo"
          n210 = Index Array(array=w524, index #1=7 ("index"), index #2=1 ("index")) -> (element #1=w519:u8, element #2=w520:u8)
          n211 = case shown="Default" w519 {
            selector: w519 -> [_ w533]
            tunnel: [T2 {"type"=enum."mark", "parameter"=254.0} ("action") w541] -> w525
            tunnel: w524 -> [w530 w538]
            tunnel: [w529 w537] -> w523
            tunnel: w520 -> [_ w534]
            frame Default {
              n212 = Replace Array Subset(array=w530, new element #1=u8 1 ("new element/subarray"), index #1=0 ("index"), new element #2=u8 0 ("new element/subarray"), index #2=7 ("index")) -> (w529:u8[])
            }
            frame 0..5 {
              n213 = Increment(x=w533) -> (x+1=w535:u8)
              n214 = call-poly "az_to_rad.vi"("az"=w534) -> ("rad"=w539:dbl)
              n215 = Replace Array Subset(array=w538, new element=w535, index=7) -> (w537:u8[])
              n216 = Bundle By Name(cluster=T2 {"type"=enum."move", "parameter"=0.0} ("action"), "parameter"=w539) -> (w541:T2)
            }
          }
        }
        frame 13 {
          # "Ranger without cargo"
          n217 = Index Array(array=w547, index #1=7 ("index"), index #2=1 ("index")) -> (element #1=w542:u8, element #2=w543:u8)
          n218 = case shown="0, 1" w542 {
            selector: w542 -> [_ w556]
            tunnel: [T2 {"type"=enum."mark", "parameter"=254.0} ("action") w564] -> w548
            tunnel: w547 -> [w553 w561]
            tunnel: [w552 w560] -> w546
            tunnel: w543 -> [_ w557]
            frame Default {
              n219 = Replace Array Subset(array=w553, new element #1=u8 7 ("new element/subarray"), index #1=0 ("index"), new element #2=u8 0 ("new element/subarray"), index #2=7 ("index")) -> (w552:u8[])
            }
            frame 0, 1 {
              n220 = Increment(x=w556) -> (x+1=w558:u8)
              n221 = call-poly "az_to_rad.vi"("az"=w557) -> ("rad"=w562:dbl)
              n222 = Replace Array Subset(array=w561, new element=w558, index=7) -> (w560:u8[])
              n223 = Bundle By Name(cluster=T2 {"type"=enum."move", "parameter"=0.0} ("action"), "parameter"=w562) -> (w564:T2)
            }
          }
        }
        frame 71 {
          # "Ranger with cargo"
          n224 = call "mark_volume.vi"("element"=T6 99, "marksArray"=w568) -> ("volume"=w567:T7)  [unwired: 9 in]
          n225 = Equal?(x=w574, y=anthillType_enum."own") -> (x = y?=w572:bool)
          n226 = Greater Than 0?(x=w567) -> (x > 0?=w566:bool)
          n227 = And(x=w572, y=w566) -> (x .and. y?=w571:bool)
          n228 = case shown="True" w571 {
            tunnel: [w580 w587] -> w575
            tunnel: w568 -> [_ w582]
            tunnel: w570 -> [w576 w585]
            tunnel: [w576 w583] -> w565
            frame False {
              # "Not at home"
              n229 = Index Array(array=w576, index=1) -> (element=w577:u8)
              n230 = call-poly "az_to_rad.vi"("az"=w577) -> ("rad"=w579:dbl)
              n231 = Bundle By Name(cluster=T2 {"type"=enum."move", "parameter"=0.0} ("action"), "parameter"=w579) -> (w580:T2)
            }
            frame True {
              # "At home"
              n232 = Index Array(array=w585, index=1) -> (element=w584:u8)
              n233 = for {
                tunnel: w582 -> [w605] mode=indexing
                tunnel: w584 -> [w599]
                tunnel: [w598] -> w588
                stop <- w598 stop-if-true
                n234 = Unbundle By Name(w605) -> ("value"=w600:T6)
                n235 = Max & Min(x=w599, y=w600) -> (max(x,y)=w604:T6, min(x,y)=w603:u8)
                n236 = Subtract(x=w604, y=w603) -> (x-y=w602:T6)
                n237 = Less?(x=w602, y=T6 1) -> (x < y?=w598:bool)
              }
              n238 = case shown="False" w588 {
                tunnel: [w593 T2 {"type"=enum."put", "parameter"=255.0} ("action")] -> w587
                tunnel: w584 -> [w590 w596]
                tunnel: w585 -> [_ _]
                tunnel: [w589 w595] -> w583
                frame False {
                  w591 = 0 ("index")
                  n239 = Bundle By Name(cluster=T2 {"type"=enum."mark", "parameter"=0.0} ("action"), "parameter"=w590) -> (w593:T2)
                  n240 = Build Array(w591, w590, w591, w591, w591, w591, w591, w591, w591) -> (w589:i32[])
                }
                frame True {
                  w594 = 0 ("index")
                  n241 = Build Array(w594, w596, w594, w594, w594, w594, w594, w594, w594) -> (w595:i32[])
                }
              }
            }
          }
        }
        frame 76 {
          # "Expirienced ranger to foodHeap"
          n242 = call "mark_volume.vi"("element"=T6 254, "marksArray"=w608) -> ("volume"=w606:T7)  [unwired: 9 in]
          n243 = case shown="1001.." w606 {
            tunnel: [w615 w623 w628] -> w609
            tunnel: w614 -> [w615 w624 w629]
            tunnel: w613 -> [_ _ _]
            tunnel: [w619 T2 {"type"=enum."mark", "parameter"=254.0} ("action") T2 {"type"=enum."take", "parameter"=254.0} ("action")] -> w612
            tunnel: w611 -> [_ _ _]
            tunnel: w610 -> [_ _ _]
            frame 0, Default {
              # "Didn't get to foodHeap"
              n244 = Index Array(array=w615, index=1) -> (element=w616:u8)
              n245 = call-poly "az_to_rad.vi"("az"=w616) -> ("rad"=w618:dbl)
              n246 = Bundle By Name(cluster=T2 {"type"=enum."move", "parameter"=0.0} ("action"), "parameter"=w618) -> (w619:T2)
            }
            frame 1..1000 {
              # "Got to foodHeap"
              n247 = Replace Array Subset(array=w624, new element=u8 7 ("new element/subarray"), index=0) -> (w623:u8[])
            }
            frame 1001.. {
              # "Got to foodHeap"
              n248 = Replace Array Subset(array=w629, new element=u8 7 ("new element/subarray"), index=0) -> (w628:u8[])
            }
          }
        }
        frame 77 {
          # "Expirienced ranger from foodHeap"
          n249 = call "mark_volume.vi"("element"=T6 99, "marksArray"=w632) -> ("volume"=w634:T7)  [unwired: 9 in]
          n250 = Equal?(x=w639, y=anthillType_enum."own") -> (x = y?=w640:bool)
          n251 = Greater Than 0?(x=w634) -> (x > 0?=w633:bool)
          n252 = And(x=w640, y=w633) -> (x .and. y?=w636:bool)
          n253 = case shown="True" w636 {
            tunnel: [w646 w651] -> w637
            tunnel: w638 -> [w642 w650]
            tunnel: [w642 w648] -> w631
            frame False {
              # "Not at home"
              n254 = Index Array(array=w642, index=1) -> (element=w643:u8)
              n255 = call-poly "az_to_rad.vi"("az"=w643) -> ("rad"=w645:dbl)
              n256 = Bundle By Name(cluster=T2 {"type"=enum."move", "parameter"=0.0} ("action"), "parameter"=w645) -> (w646:T2)
            }
            frame True {
              # "At home"
              n257 = Index Array(array=w650, index=6) -> (element=w649:u8)
              n258 = case shown="0" w649 {
                selector: w649 -> [w654 _]
                tunnel: [w664 T2 {"type"=enum."empty", "parameter"=0.0} ("action")] -> w651
                tunnel: w650 -> [w655 w669]
                tunnel: [w653 w666] -> w648
                frame Default {
                  n259 = Bundle By Name(cluster=T2 {"type"=enum."mark", "parameter"=0.0} ("action"), "parameter"=w654) -> (w664:T2)
                  n260 = Replace Array Subset(array=w655, new element #1=u8 8 ("new element/subarray"), index #1=0 ("index"), new element #2=u8 0 ("new element/subarray"), index #2=4 ("index"), new element #3=u8 0 ("new element/subarray"), index #3=5 ("index"), new element #4=u8 0 ("new element/subarray"), index #4=6 ("index")) -> (w653:u8[])
                }
                frame 0 {
                  n261 = Replace Array Subset(array=w669, new element #1=u8 8 ("new element/subarray"), index #1=0 ("index"), new element #2=u8 0 ("new element/subarray"), index #2=4 ("index"), new element #3=u8 0 ("new element/subarray"), index #3=5 ("index"), new element #4=u8 0 ("new element/subarray"), index #4=6 ("index")) -> (w666:u8[])
                }
              }
            }
          }
        }
        frame 100 {
          # "Administrator"
          n262 = for {
            tunnel: w678 -> [w689] mode=indexing
            shift-right: [w686] -> w677
            shift-left: w679 -> [w687]
            n263 = Unbundle By Name(w689) -> ("value"=w688:T6)
            n264 = case shown="60..89" w688 {
              selector: w688 -> [_ w693 w698 w707]
              tunnel: w687 -> [w690 w695 w702 w711]
              tunnel: [w690 w694 w699 w708] -> w686
              frame Default {
              }
              frame 0..29 {
                w692 = T6 0 ("element")
                n265 = Build Array(w693, w692, w692) -> (w691:T6[])
                n266 = Insert Into Array(array=w695, new element=w691) -> (w694:i32[][])  [unwired: 2 in]
              }
              frame 30..59 {
                n267 = Index Array(array=w702, index (col)=0 ("disabled index (col)")) -> (element=w703:i32[])  [unwired: 1 in]
                n268 = Subtract(x=w698, y=T6 30) -> (x-y=w696:T6)
                n269 = Search 1D Array(1D array=w703, element=w696) -> (index of element=w701:i32)  [unwired: 1 in]
                n270 = Replace Array Subset(array=w702, new element=w696, index (row)=w701, index (col)=2 ("disabled index (col)")) -> (w699:i32[][])
              }
              frame 60..89 {
                n271 = Index Array(array=w711, index (col)=0 ("disabled index (col)")) -> (element=w712:i32[])  [unwired: 1 in]
                n272 = Subtract(x=w707, y=T6 60) -> (x-y=w705:T6)
                n273 = Search 1D Array(1D array=w712, element=w705) -> (index of element=w710:i32)  [unwired: 1 in]
                n274 = Replace Array Subset(array=w711, new element=w705, index (row)=w710, index (col)=1 ("disabled index (col)")) -> (w708:i32[][])
              }
            }
          }
          "Array" <- w677
          n275 = call "mark_volume.vi"("element"=T6 99, "marksArray"=w678) -> ("volume"=w681:T7)  [unwired: 9 in]
          n276 = Greater Than 0?(x=w681) -> (x > 0?=w680:bool)
          n277 = case shown="True" w680 {
            tunnel: [w715 w731] -> w685
            tunnel: w684 -> [w716 w730]
            tunnel: [w716 w723] -> w683
            tunnel: w678 -> [w717 w722]
            frame False {
              n278 = call "mark_volume.vi"("element"=T6 123, "marksArray"=w717) -> ("volume"=w718:T7)  [unwired: 9 in]
              n279 = Greater Than 0?(x=w718) -> (x > 0?=w714:bool)
              n280 = case shown="False" w714 {
                tunnel: [T2 {"type"=enum."mark", "parameter"=98.0} ("action") T2 {"type"=enum."mark", "parameter"=99.0} ("action")] -> w715
                frame False {
                }
                frame True {
                }
              }
            }
            frame True {
              n281 = for {
                tunnel: w722 -> [w757] mode=indexing
                shift-right: [w755] -> w723
                shift-left: w730 -> [w756]
                n282 = Unbundle By Name(w757) -> ("value"=w754:T6)
                n283 = case shown="30..59" w754 {
                  selector: w754 -> [_ w759 w774]
                  tunnel: w756 -> [w758 w762 w776]
                  tunnel: [w758 w761 w775] -> w755
                  frame Default {
                  }
                  frame 0..29 {
                    n284 = Add(x=w759, y=T6 30) -> (x+y=w767:T6)
                    n285 = Search 1D Array(1D array=w762, element=w759) -> (index of element=w768:i32)  [unwired: 1 in]
                    n286 = Search 1D Array(1D array=w762, element=w767) -> (index of element=w764:i32)  [unwired: 1 in]
                    n287 = Less Than 0?(x=w768) -> (x < 0?=w765:bool)
                    n288 = Less Than 0?(x=w764) -> (x < 0?=w763:bool)
                    n289 = And(x=w765, y=w763) -> (x .and. y?=w760:bool)
                    n290 = case shown="True" w760 {
                      tunnel: w762 -> [w769 w772]
                      tunnel: [w769 w771] -> w761
                      tunnel: w759 -> [_ w770]
                      frame False {
                      }
                      frame True {
                        n291 = Insert Into Array(array=w772, new element=w770) -> (w771:u8[])  [unwired: 1 in]
                      }
                    }
                  }
                  frame 30..59 {
                    n292 = Search 1D Array(1D array=w776, element=w774) -> (index of element=w777:i32)  [unwired: 1 in]
                    n293 = Less Than 0?(x=w777) -> (x < 0?=w773:bool)
                    n294 = case shown="True" w773 {
                      tunnel: w776 -> [w778 w783]
                      tunnel: [w778 w781] -> w775
                      tunnel: w774 -> [_ w780]
                      frame False {
                      }
                      frame True {
                        n295 = Subtract(x=w780, y=T6 30) -> (x-y=w785:T6)
                        n296 = Insert Into Array(array=w783, new element=w780) -> (w782:u8[])  [unwired: 1 in]
                        n297 = Search 1D Array(1D array=w783, element=w785) -> (index of element=w779:i32)  [unwired: 1 in]
                        n298 = Delete From Array(array=w782, index=w779) -> (array with subset deleted=w781:u8[])  [unwired: 1 in, 1 out]
                      }
                    }
                  }
                }
              }
              n299 = for {
                tunnel: w723 -> [w751] mode=indexing
                tunnel: [w751] -> w729 if=w750
                tunnel: [w750] -> w724
                stop <- w750 stop-if-true
                n300 = In Range and Coerce(upper limit=u8 29, x=w751, lower limit=u8 0) -> (In Range?=w750:bool)  [unwired: 1 out]
              }
              n301 = call "mark_volume.vi"("element"=T6 99, "marksArray"=w722) -> ("volume"=w728:T7)  [unwired: 9 in]
              n302 = Less Or Equal?(x=w728, y=T7 1000) -> (x <= y?=w725:bool)
              n303 = case shown="False" w725 {
                tunnel: [w735 T2 {"type"=enum."mark", "parameter"=99.0} ("action")] -> w731
                tunnel: w729 -> [w733 _]
                tunnel: w722 -> [w734 _]
                tunnel: w724 -> [w732 _]
                frame False {
                  n304 = case shown="True" w732 {
                    tunnel: [T2 {"type"=enum."empty", "parameter"=0.0} ("action") w744] -> w735
                    tunnel: w734 -> [_ w740]
                    tunnel: w733 -> [_ w739]
                    frame False {
                    }
                    frame True {
                      n305 = Add(x=w739, y=u8 60) -> (x+y=w737:u8)
                      n306 = call "mark_volume.vi"("element"=w737, "marksArray"=w740) -> ("volume"=w743:T7)  [unwired: 9 in]
                      n307 = Less Or Equal?(x=w743, y=T7 1000) -> (x <= y?=w741:bool)
                      n308 = case shown="False" w741 {
                        tunnel: [T2 {"type"=enum."empty", "parameter"=0.0} ("action") w748] -> w744
                        tunnel: w737 -> [_ w747]
                        frame False {
                        }
                        frame True {
                          n309 = Bundle By Name(cluster=T2 {"type"=enum."mark", "parameter"=0.0} ("action"), "parameter"=w747) -> (w748:T2)
                        }
                      }
                    }
                  }
                }
                frame True {
                }
              }
            }
          }
        }
      }
    }
    frame True {
      # "Ant's memory is empty"
      n310 = Empty Array?(array=w786) -> (empty?=w789:bool)
      n311 = case shown="False" w789 {
        tunnel: [w798 w834] -> w790
        tunnel: [w797 w832] -> w788
        tunnel: w786 -> [w793 _]
        tunnel: w787 -> [w796 _]
        tunnel: w786 -> [w795 _]
        frame False {
          n312 = call "mark_with_max_volume_min.vi"("marksArray"=w793) -> ("markValue"=w792:T5)
          n313 = Unbundle By Name(w792) -> ("value"=w794:T6)
          n314 = case shown="99" w794 {
            tunnel: [T2 {"type"=enum."empty", "parameter"=0.0} ("action") w807 w830] -> w798
            tunnel: [w801 w806 w824] -> w797
            tunnel: w796 -> [_ _ w824]
            tunnel: w795 -> [_ w805 w822]
            frame 98 {
              n315 = Build Array(10 ("index (row)")) -> (w801:i32[])
            }
            frame 99 {
              n316 = call "mark_with_max_volume.vi"("marksArray"=w805) -> ("markValue"=w804:T5)
              n317 = Unbundle By Name(w804) -> ("value"=w803:T6)
              n318 = Increment(x=w803) -> (x+1=w802:T6)
              n319 = case shown="100..129" w802 {
                selector: w802 -> [w809 _]
                tunnel: [w813 w819] -> w807
                tunnel: [w811 w817] -> w806
                frame 100..129 {
                  w808 = T6 0 ("element")
                  # "Ant became a ranger"
                  n320 = Subtract(x=w809, y=T6 100) -> (x-y=w810:T6)
                  n321 = Build Array(w808, w810, w808, w808, w808, w808, w808, w808, w808) -> (w811:T6[])
                  n322 = Bundle By Name(cluster=T2 {"type"=enum."mark", "parameter"=0.0} ("action"), "parameter"=w809) -> (w813:T2)
                }
                frame Default {
                  w815 = T6 0 ("element")
                  # "Ant became an ant-on-duty"
                  n323 = Build Array(T6 2 ("element"), w815, w815, w815, w815, w815, w815, w815, w815) -> (w817:T6[])
                  n324 = Bundle By Name(cluster=T2 {"type"=enum."mark", "parameter"=0.0} ("action"), "parameter"=T6 130 ("lower limit")) -> (w819:T2)
                }
              }
            }
            frame Default {
              n325 = Delete From Array(array=w822) -> (deleted portion=w823:T5)  [unwired: 2 in, 1 out]
              n326 = Unbundle By Name(w823) -> ("value"=w821:T6)
              n327 = Increment(x=w821) -> (x+1=w828:T6)
              n328 = In Range and Coerce(upper limit=T6 200, x=w828, lower limit=T6 100) -> (coerced(x)=w827:T6)  [unwired: 1 out]
              n329 = Bundle By Name(cluster=T2 {"type"=enum."mark", "parameter"=0.0} ("action"), "parameter"=w827) -> (w830:T2)
            }
          }
        }
        frame True {
          w831 = T6 100 ("element")
          n330 = Build Array(w831) -> (w832:T6[])
          n331 = Bundle By Name(cluster=T2 {"type"=enum."mark", "parameter"=0.0} ("action"), "parameter"=w831) -> (w834:T2)
        }
      }
    }
  }
  "error out" <- w21
  "action" <- w20
  n332 = call "memory_set.vi"("memory"=w4, "ant_base in"=w5) -> ("ant_base out"=→"Igor out":refnum<class "Igor.lvclass">)  [unwired: 8 in, 1 out]
